vi "Demo_1.vi"() -> ()   [LabVIEW 2014]
uses:
  TypeDefs/Boolean&NumericData.ctl
  <vilib>/Utility/miscctls.llb/LVRowAndColumnTypeDef.ctl
  TypeDefs/LogicParsedExpression.ctl
  TypeDefs/Variable State.ctl
  <vilib>/Utility/file.llb/Read From Spreadsheet File (string).vi
panel:
  in  "Start":bool
  in  "Open Cfg":bool
  in  "Save Cfg":bool
  in  "New Cfg":bool
  in  "Secuencia de Ciclo de Medición":string[][](table)
  in  "Close Seq":bool
  out "Tab Control":enum32{"HOME", "CONFIG.", "CICLO"}(tab)
  out "Editor de Programas Ind":string[][](table)
  in  "Editor de Programas Ctl":string[][](table)
  in  "Diseño":string
  in  "Cód. Prog.":i32
  in  "Autor":string
  in  "Nombre Programa":string
  in  "Descripción":string
  in  "Pieza":i32
  in  "Operación":i32
  in  "Tipo de Programa":enum16{"CAP", "Engranometro"}(ring)
  in  "Secuencia Ciclo":bool
  in  "Secuencia de Ciclo de Medición":string[][](table)
  out "Estado":string
  in  "Angle":sgl(knob) scale=-720.0..720.0
  in  "Cluster":T1
  in  "CICLO":bool
  in  "CONFIG.":bool
  in  "HOME":bool
  in  "Ruta de Sec":path
  in  "Logic Variable Data":T2
  out "error out":errorcluster
  in  "error in (no error)":errorcluster
  # "DEMO Modulo Secuencial"
  # "Programa de Medición"
  # "Instrucciones de Uso"
  # "- Panel Configuración-\n1. Crear Nuevo Configuración o Abrir una ya existente \n\n- Panel Driver -\n1. En la lista desplegable se pueden visualizar y selecciona\n2. Una vez seleccionado un Proceso se puede \n3. Para acceder a su panel de configuración \n\n- CONECTAR -\n1. Una vez definida la configuración de Drivers que uno desea, al presionar \"Conectar >\" se establec\n\n- Panel Dispositivos Conectados -\n1. Una vez conectados los dispositivos se podrá seleccionar cada Dispositivo que esté \n\n- DESCONECTAR -\n1. Una vez que desee terminar con la adquisición, debe presionar \"Desconectar\nsino la aplicación devolverá error."
  # "Editor de Programa de Medición"
  # "Secuencia de Ciclo de Medición"
  # "Entradas Numeradas"
  # "Encoder"
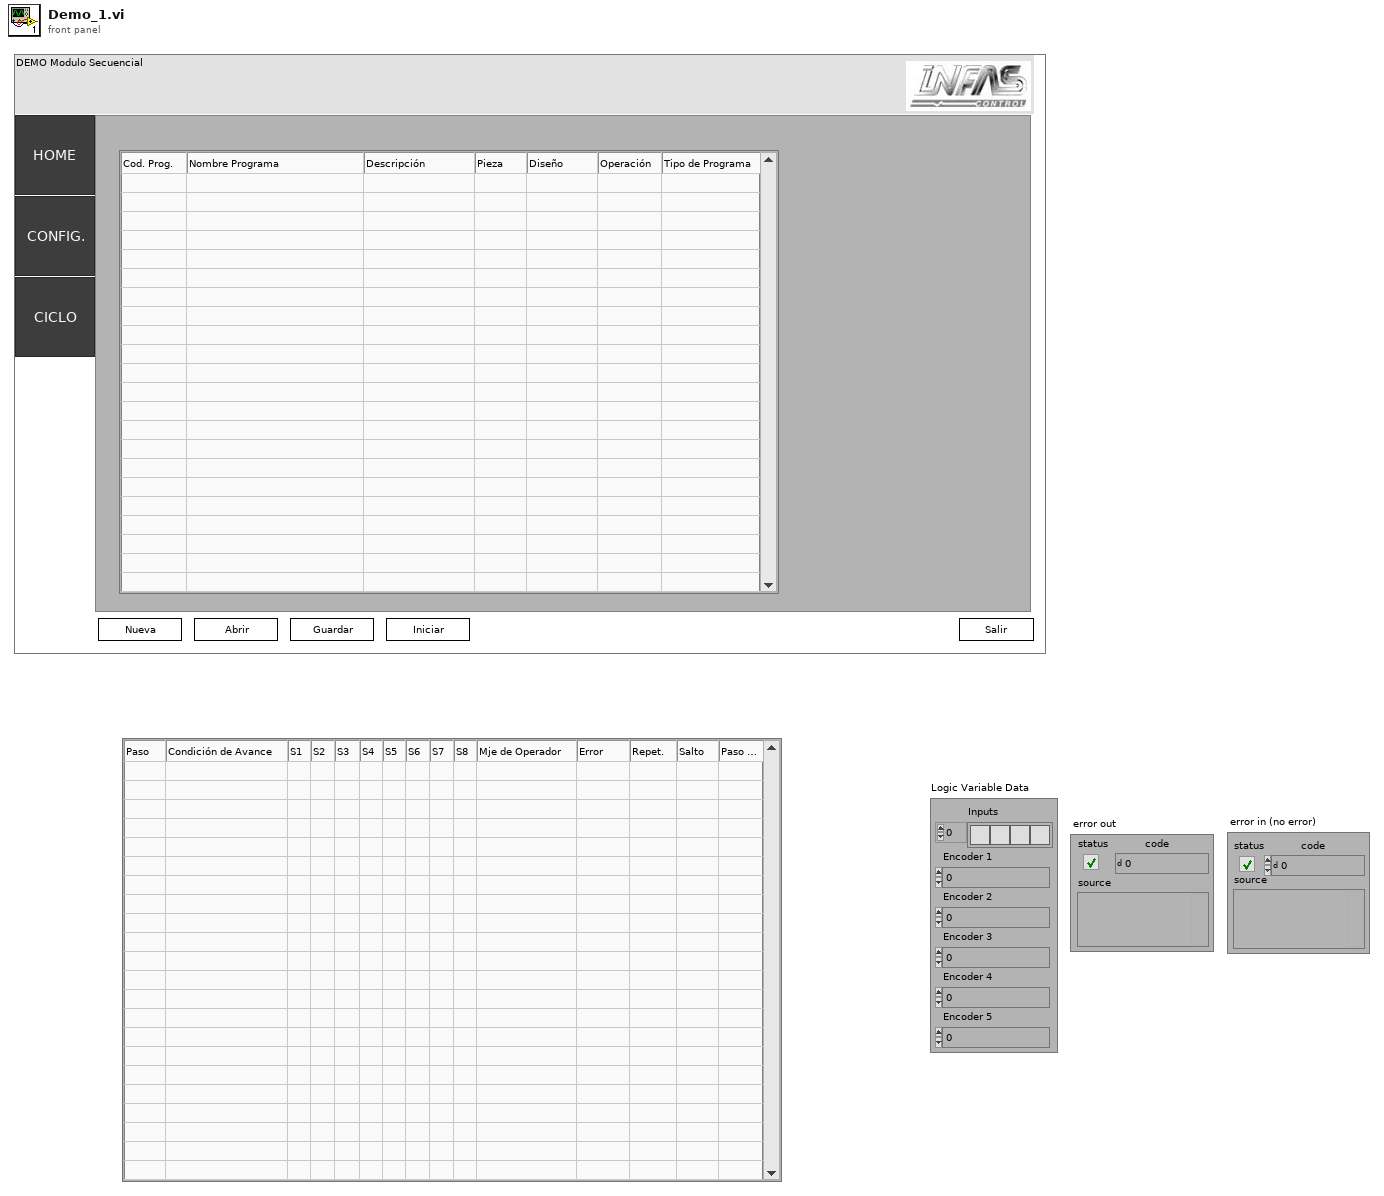
[diagram p1: front panel]
types:
  T1 = cluster{"Boolean 2":bool, "Boolean 1":bool, "Boolean 3":bool, "Boolean 4":bool, "Boolean 5":bool, "Boolean 6":bool, "Boolean 7":bool, "Boolean 8":bool, "Boolean 9":bool, "Boolean 10":bool, "Boolean 11":bool, "Boolean 12":bool}
  T2 = typedef "Boolean&NumericData.ctl" = cluster{"Inputs":bool[], "Encoder 1":sgl, "Encoder 2":sgl, "Encoder 3":sgl, "Encoder 4":sgl, "Encoder 5":sgl}
  T3 = typedef "Variable State.ctl" = cluster{"I":bool[], "P":bool[], "N":bool[], "T":bool[], "X":bool[], "Timer":u32[], "Wait":u32, "Wait?":bool}
  T4 = typedef "LogicParsedExpression.ctl" = cluster{"RPN ":string[], "Variables":string[], "Ctes":string[], "Formula":string, "Message":string}
  T5 = typedef "LVRowAndColumnTypeDef.ctl" = cluster{"Row":i32, "Column":i32}
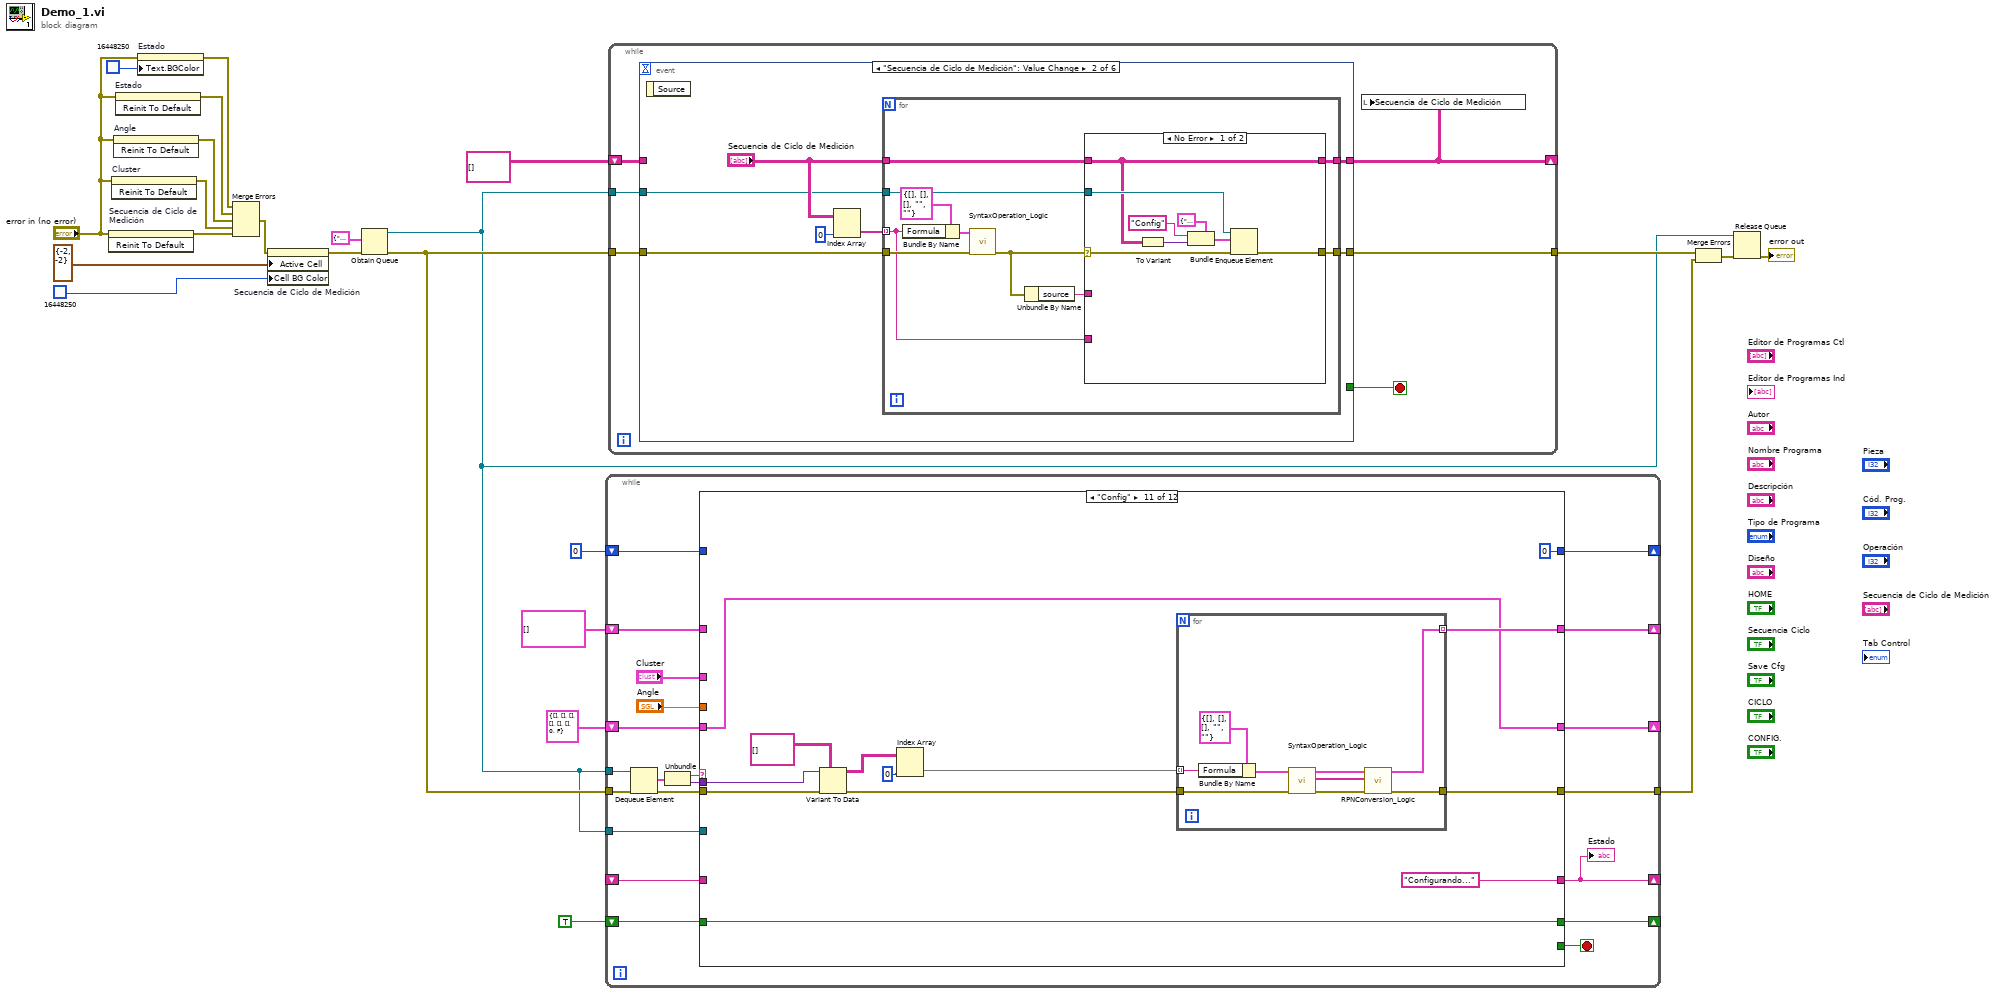
[diagram p0: block diagram]
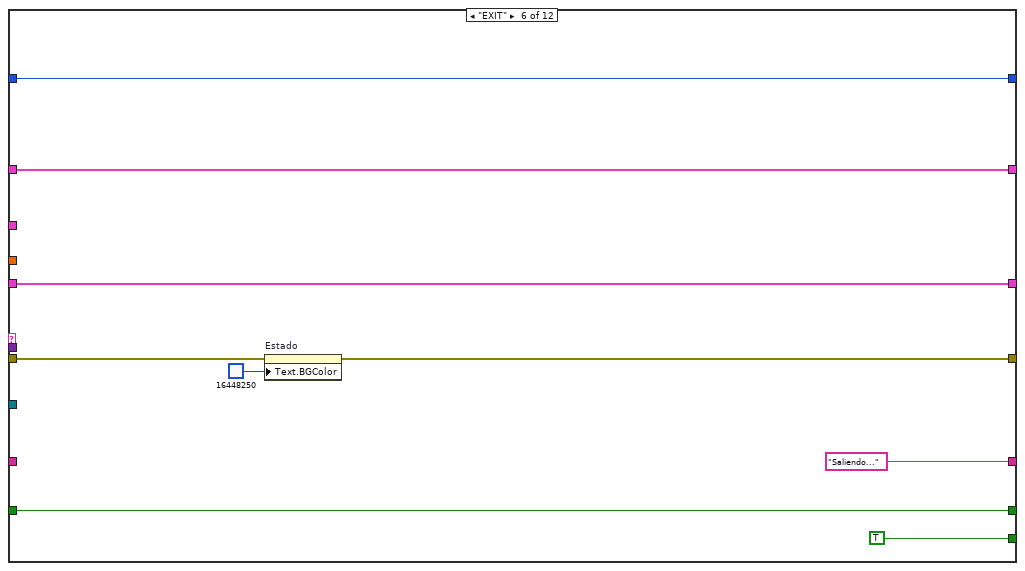
[diagram p7: hidden frame]
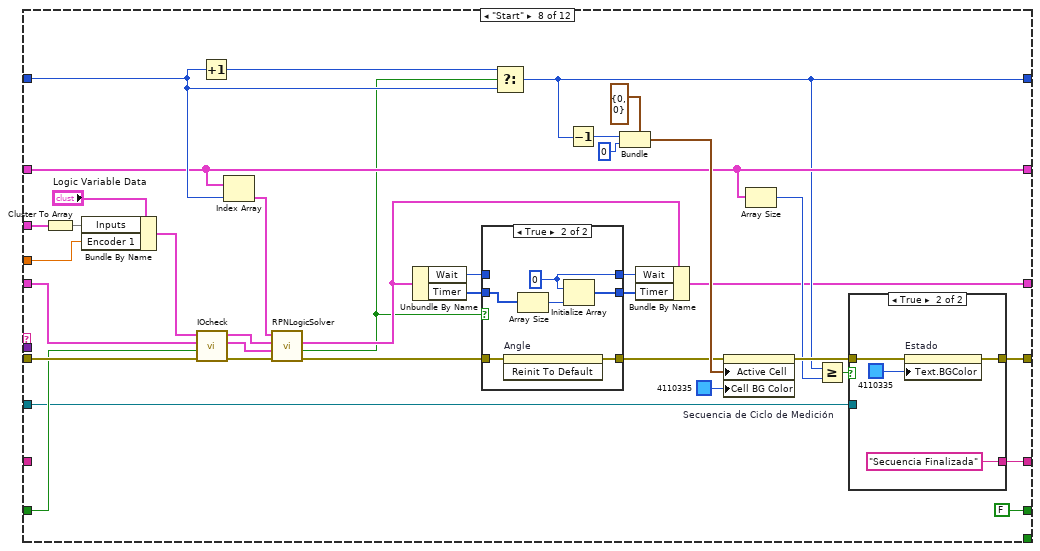
[diagram p9: hidden frame]
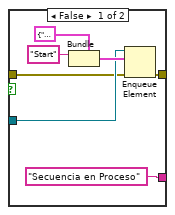
[diagram p11: hidden frame]
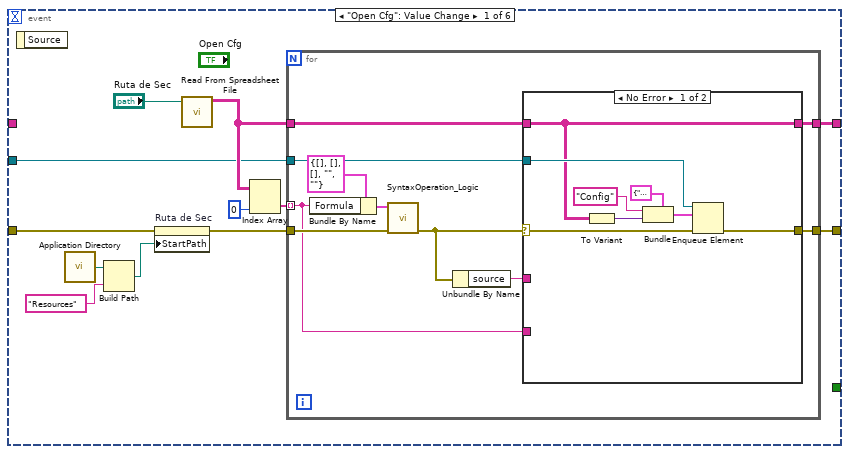
[diagram p15: hidden frame]
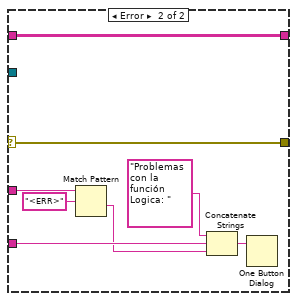
[diagram p16: hidden frame]
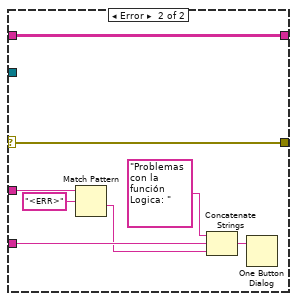
[diagram p17: hidden frame]
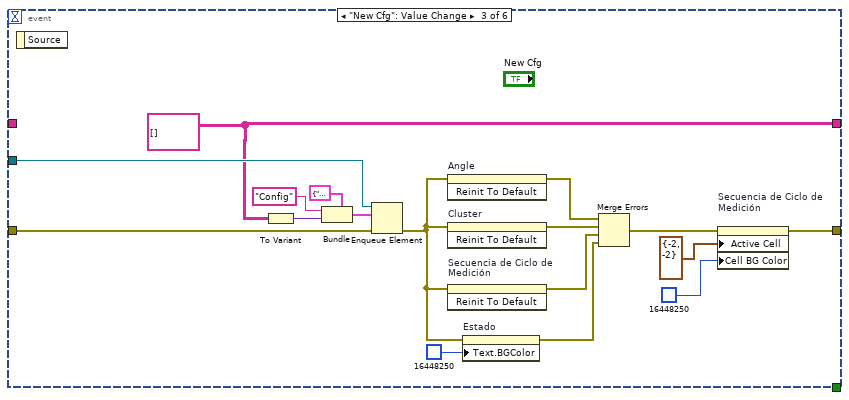
[diagram p18: hidden frame]
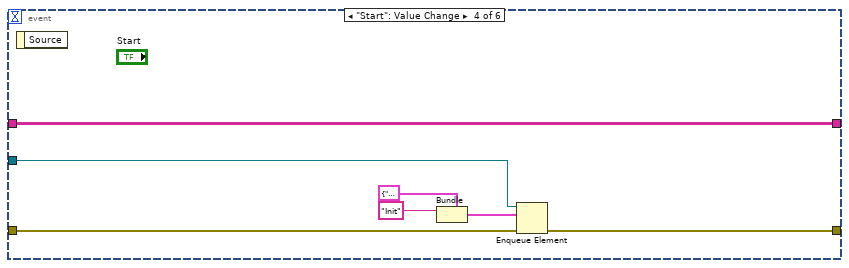
[diagram p19: hidden frame]
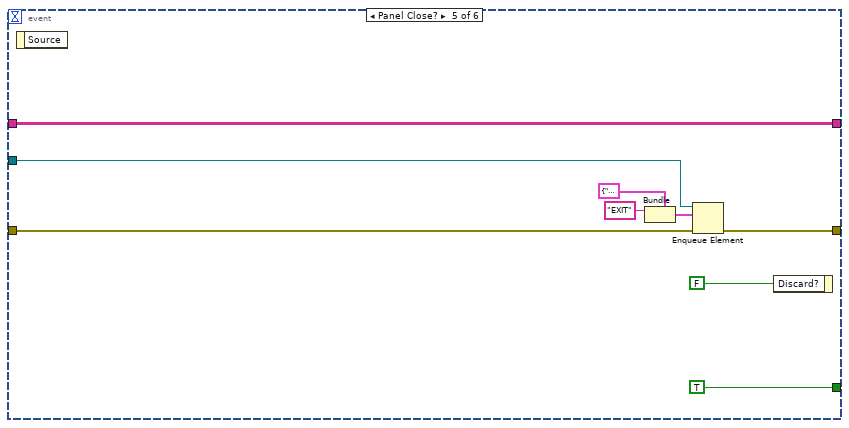
[diagram p20: hidden frame]
diagram:
  n1 = invoke on="Secuencia de Ciclo de Medición" class="Tbl (strict)" method="Reinit To Default"(error in="error in (no error)") -> (error out=w13:errorcluster)  [unwired: 2 in, 2 out]
  n2 = invoke on="Cluster" class="Clust (strict)" method="Reinit To Default"(error in="error in (no error)") -> (error out=w11:errorcluster)  [unwired: 2 in, 2 out]
  n3 = invoke on="Angle" class="Knob (strict)" method="Reinit To Default"(error in="error in (no error)") -> (error out=w5:errorcluster)  [unwired: 2 in, 2 out]
  n4 = invoke on="Estado" class="Str" method="Reinit To Default"(error in="error in (no error)") -> (error out=w4:errorcluster)  [unwired: 2 in, 2 out]
  n5 = property on="Estado" class="Str"(error in="error in (no error)", "Text.BGColor"=u32 16448250) -> (error out=w1:errorcluster)  [unwired: 1 in, 1 out]
  n6 = Merge Errors(w1, w4, w5, w11, w13) -> (w12:errorcluster)
  n7 = property on="Secuencia de Ciclo de Medición" class="Tbl (strict)"(error in=w12, "Active Cell"=T5 {"Row"=-2, "Column"=-2} ("Active Cell:Active Cell"), "Cell BG Color"=u32 16448250) -> (error out=w19:errorcluster)  [unwired: 1 in, 1 out]
  n8 = Obtain Queue(element data type=cluster{string, variant} {"", variant}, error in (no error)=w19) -> (queue out=w6:refnum<queue>, error out=w18:errorcluster)  [unwired: 3 in, 1 out]
  n9 = while {
    tunnel: w18 -> [w43]
    tunnel: [w44] -> w16
    tunnel: w6 -> [w42]
    shift-right: [w35] -> _
    shift-left: T4[] [] -> [w36]
    shift-right: [w33] -> _
    shift-left: T3 {"I"=[], "P"=[], "N"=[], "T"=[], "X"=[], "Timer"=[], "Wait"=0, "Wait?"=FALSE} ("Variable State") -> [w34]
    shift-right: [w31] -> _
    shift-left: TRUE ("First call?") -> [w32]
    shift-right: [w30] -> _
    shift-left: 0 -> [w29]
    tunnel: w6 -> [w28]
    shift-right: [w25] -> _
    shift-left: _ -> [w24]
    stop <- w37 stop-if-true
    n10 = Dequeue Element(queue=w42, error in (no error)=w43) -> (element=w41:cluster{string, variant}, error out=w38:errorcluster)  [unwired: 1 in, 2 out]
    n11 = Unbundle(w41) -> (w40:string, w39:variant)
    n12 = case shown="\"Config\"" w40 {
      tunnel: [w47 w52 w59 w65 w71 w75 w89 w107 w149 w155 w164 w183] -> w44
      tunnel: w38 -> [w47 w52 w59 w65 w71 w76 w89 w126 w149 w155 w171 w183]
      tunnel: w39 -> [_ _ _ _ _ _ _ _ _ _ w170 _]
      tunnel: [_ _ _ _ _ TRUE _ _ _ _ _ _] -> w37
      tunnel: w36 -> [w49 w54 w61 w67 w73 w82 w88 w105 w151 w157 _ w185]
      tunnel: [w49 w54 w61 w67 w73 w82 w88 w105 w151 w157 w163 w185] -> w35
      tunnel: w34 -> [w48 w53 w60 w66 w72 w80 w87 w125 w150 w156 w161 w184]
      tunnel: [w48 w53 w60 w66 w72 w80 w87 w93 w150 w156 w161 w184] -> w33
      tunnel: w32 -> [w45 w56 w57 w63 w69 w81 w86 w124 w147 w153 w162 w181]
      tunnel: [w45 w56 w57 w63 w69 w81 w86 FALSE ("First call?") w147 w153 w162 w181] -> w31
      tunnel: [w50 w55 w62 w68 w74 w79 w85 w103 w152 w158 0 w186] -> w30
      tunnel: w29 -> [w50 w55 w62 w68 w74 w79 w85 w110 w152 w158 _ w186]
      tunnel: w28 -> [_ _ _ _ _ _ _ w109 _ _ _ _]
      tunnel: "Cluster" -> [_ _ _ _ _ _ _ w100 _ _ _ _]
      tunnel: "Angle" -> [_ _ _ _ _ _ _ w99 _ _ _ _]
      tunnel: [w46 w51 w58 w64 w70 "Saliendo..." w84 w94 w148 w154 "Configurando..." w182] -> w25
      tunnel: w24 -> [w46 w51 w58 w64 w70 _ w84 _ w148 w154 _ w182]
      frame "----LOOP----" {
        # "Bloque que adminte futuras configuraciones al inicio."
      }
      frame Default {
      }
      frame "LOAD" {
      }
      frame "INIT" {
      }
      frame "UPLOAD" {
      }
      frame "EXIT" {
        n13 = property on="Estado" class="Str"(error in=w76, "Text.BGColor"=u32 16448250) -> (error out=w75:errorcluster)  [unwired: 1 in, 1 out]
      }
      frame "----ACTION----" {
      }
      frame "Start" {
        n14 = Cluster To Array(cluster=w100) -> (array=w112:bool[])
        n15 = Bundle By Name(cluster="Logic Variable Data", "Inputs"=w112, "Encoder 1"=w99) -> (w113:T2)
        n16 = call "IOcheck.vi"("error in (no error)"=w126, "First call?"=w124, "Variable State"=w125, "Logic Variable Data"=w113) -> ("error out"=w116:errorcluster, "Variable State Out"=w117:T3, "Logic Variable Data Out"=w118:T2)  [unwired: 5 in]
        n17 = Increment(x=w110) -> (x+1=w115:i32)
        n18 = Index Array(array=w105, index=w110) -> (element=w111:T4)
        n19 = call "RPNLogicSolver.vi"("error in"=w116, "Variable State"=w117, "Logic Variable Data Out"=w118, "Logic Parsed Expression"=w111) -> ("error out"=w96:errorcluster, "Logical Operation Out"=w92:bool, "Variable State Out"=w101:T3)  [unwired: 4 in, 1 out]
        n20 = Unbundle By Name(w101) -> ("Wait"=w90:u32, "Timer"=w97:u32[])
        n21 = case shown="True" w92 {
          tunnel: [w129 w134] -> w98
          tunnel: w97 -> [w129 w133]
          tunnel: w96 -> [w128 w132]
          tunnel: [w128 w131] -> w95
          tunnel: [w127 w130] -> w91
          tunnel: w90 -> [w127 _]
          frame False {
          }
          frame True {
            w130 = u32 0 ("element")
            n22 = invoke on="Angle" class="Knob (strict)" method="Reinit To Default"(error in=w132) -> (error out=w131:errorcluster)  [unwired: 2 in, 2 out]
            n23 = Array Size(array=w133) -> (size(s)=w135:i32)
            n24 = Initialize Array(w130, w135) -> (w134:u32[])
          }
        }
        n25 = Select(t=w115, s=w92, f=w110) -> (s? t:f=w103:i32)
        n26 = Decrement(x=w103) -> (x-1=w102:i32)
        n27 = Bundle(cluster=T5 {"Row"=0, "Column"=0} ("Active Cell:Active Cell"), "Row"=w102, "Column"=0 ("Row")) -> (w119:T5)
        n28 = Bundle By Name(cluster=w101, "Wait"=w91, "Timer"=w98) -> (w93:T3)
        n29 = property on="Secuencia de Ciclo de Medición" class="Tbl (strict)"(error in=w95, "Active Cell"=w119, "Cell BG Color"=u32 4110335) -> (error out=w108:errorcluster)  [unwired: 1 in, 1 out]
        n30 = Array Size(array=w105) -> (size(s)=w104:i32)
        n31 = Greater Or Equal?(x=w103, y=w104) -> (x >= y?=w106:bool)
        n32 = case shown="True" w106 {
          tunnel: w109 -> [w139 _]
          tunnel: w108 -> [w138 w145]
          tunnel: [w137 w143] -> w107
          tunnel: ["Secuencia en Proceso" "Secuencia Finalizada"] -> w94
          frame False {
            n33 = Bundle(cluster=cluster{string, variant} {"", variant}, "Start") -> (w142:cluster{string, variant})  [unwired: 1 in]
            n34 = Enqueue Element(queue=w139, element=w142, error in (no error)=w138) -> (error out=w137:errorcluster)  [unwired: 1 in, 2 out]
          }
          frame True {
            n35 = property on="Estado" class="Str"(error in=w145, "Text.BGColor"=u32 4110335) -> (error out=w143:errorcluster)  [unwired: 1 in, 1 out]
          }
        }
      }
      frame "----UTILITY----" {
      }
      frame "Config:Set" {
      }
      frame "Config" {
        n36 = Variant To Data(error in=w171, type=string[][] [] ("Secuencia de Ciclo de Medición"), Variant=w170) -> (data=w167:string[][], error out=w165:errorcluster)
        n37 = Index Array(array=w167, index (col)=0 ("index (row)")) -> (element=w166:string[])  [unwired: 1 in]
        n38 = for {
          tunnel: w166 -> [w176] mode=indexing
          tunnel: w165 -> [w175]
          tunnel: [w174] -> w164
          tunnel: [w173] -> w163 mode=indexing
          n39 = Bundle By Name(cluster=T4 {"RPN "=[], "Variables"=[], "Ctes"=[], "Formula"="", "Message"=""} ("Logical Parsed Expression Out"), "Formula"=w176) -> (w177:T4)
          n40 = call "SyntaxOperation_Logic.vi"("error in (no error)"=w175, "Logical Parsed Expression"=w177) -> ("error out"=w178:errorcluster, "Token"=w180:string[], "Logical Parsed Expression Out"=w179:T4)  [unwired: 6 in, 1 out]
          n41 = call "RPNConversion_Logic.vi"("error in"=w178, "Token"=w180, "Logical Parsed Expression"=w179) -> ("error out"=w174:errorcluster, "Logical Parsed Expression Out"=w173:T4)  [unwired: 7 in]
        }
      }
      frame "Config:Get" {
      }
    }
    "Estado" <- w25
  }
  n42 = while {
    tunnel: w18 -> [w191]
    tunnel: [w190] -> w15
    shift-right: [w187] -> _
    shift-left: string[][] [] ("Secuencia de Ciclo de Medición") -> [w192]
    tunnel: w6 -> [w188]
    stop <- w189 stop-if-true
    n43 = event shown="[1] \"Secuencia de Ciclo de Medición\": Value Change" {
      selector: _ -> [_ _ _ _ _ _]
      dyn-events: _ -> [_ _ _ _ _ _]
      timeout: _ -> [_ _ _ _ _ _]
      tunnel: w192 -> [_ _ _ w287 w296 w303]
      tunnel: w191 -> [w194 w233 w275 w284 w292 w299]
      tunnel: [w201 w234 w267 w283 w291 w298] -> w190
      tunnel: [w202 w231 w274 w287 w296 w303] -> w187
      tunnel: [_ _ _ _ TRUE ("Discard?") TRUE ("Discard?")] -> w189
      tunnel: w188 -> [w199 w232 w276 w282 w288 w297]
      event "Open Cfg": Value Change {
        n44 = event-data() -> ()  [unwired: 1 in, 1 out]
        n45 = call <vilib>:"Application Directory.vi"() -> ("Application Directory"=w197:path)
        n46 = Build Path(base path=w197, name or relative path="Resources") -> (appended path=w195:path)
        n47 = property on="Ruta de Sec" class="Path"(error in=w194, "StartPath"=w195) -> (error out=w193:errorcluster)  [unwired: 1 in, 1 out]
        n48 = call-poly <vilib>:"Read From Spreadsheet File.vi"("file path (dialog if empty)"="Ruta de Sec") -> ("all rows"=w200:string[][])  [unwired: 6 in, 4 out]
        n49 = Index Array(array=w200, index (col)=0 ("disabled index (col)")) -> (element=w203:string[])  [unwired: 1 in]
        n50 = for {
          tunnel: w203 -> [w205] mode=indexing
          tunnel: w200 -> [w213]
          tunnel: [w212] -> w201
          tunnel: w193 -> [w211]
          tunnel: w199 -> [w210]
          tunnel: [w209] -> w202
          n51 = Bundle By Name(cluster=T4 {"RPN "=[], "Variables"=[], "Ctes"=[], "Formula"="", "Message"=""} ("Logical Parsed Expression"), "Formula"=w205) -> (w206:T4)
          n52 = call "SyntaxOperation_Logic.vi"("error in (no error)"=w211, "Logical Parsed Expression"=w206) -> ("error out"=w208:errorcluster)  [unwired: 6 in, 3 out]
          n53 = Unbundle By Name(w208) -> ("source"=w207:string)
          n54 = case shown="No Error" w208 {
            selector: w208 -> [w215 w230]
            tunnel: w213 -> [w216 w229]
            tunnel: [w218 w230] -> w212
            tunnel: w210 -> [w217 _]
            tunnel: [w216 w229] -> w209
            tunnel: w207 -> [_ w228]
            tunnel: w205 -> [_ w224]
            frame No Error {
              n55 = To Variant(anything=w216) -> (Variant=w221:variant)
              n56 = Bundle(cluster=cluster{string, variant} {"", variant}, "Config", w221) -> (w219:cluster{string, variant})
              n57 = Enqueue Element(queue=w217, element=w219, error in (no error)=w215) -> (error out=w218:errorcluster)  [unwired: 1 in, 2 out]
            }
            frame Error {
              n58 = Match Pattern(string=w228, regular expression="<ERR>") -> (after substring=w223:string)  [unwired: 1 in, 3 out]
              n59 = Concatenate Strings("Problemas con la función Logica: " ("string"), w224, w223) -> (w226:string)
              n60 = One Button Dialog(message=w226) -> ()  [unwired: 1 in, 1 out]
            }
          }
        }
      }
      event "Secuencia de Ciclo de Medición": Value Change {
        n61 = event-data() -> ()  [unwired: 1 in, 1 out]
        n62 = Index Array(array="Secuencia de Ciclo de Medición", index (col)=0 ("disabled index (col)")) -> (element=w236:string[])  [unwired: 1 in]
        n63 = for {
          tunnel: w236 -> [w238] mode=indexing
          tunnel: "Secuencia de Ciclo de Medición" -> [w246]
          tunnel: [w245] -> w234
          tunnel: w233 -> [w244]
          tunnel: w232 -> [w243]
          tunnel: [w242] -> w231
          n64 = Bundle By Name(cluster=T4 {"RPN "=[], "Variables"=[], "Ctes"=[], "Formula"="", "Message"=""} ("Logical Parsed Expression"), "Formula"=w238) -> (w239:T4)
          n65 = call "SyntaxOperation_Logic.vi"("error in (no error)"=w244, "Logical Parsed Expression"=w239) -> ("error out"=w241:errorcluster)  [unwired: 6 in, 3 out]
          n66 = Unbundle By Name(w241) -> ("source"=w240:string)
          n67 = case shown="No Error" w241 {
            selector: w241 -> [w248 w263]
            tunnel: w246 -> [w249 w262]
            tunnel: [w251 w263] -> w245
            tunnel: w243 -> [w250 _]
            tunnel: [w249 w262] -> w242
            tunnel: w240 -> [_ w261]
            tunnel: w238 -> [_ w257]
            frame No Error {
              n68 = To Variant(anything=w249) -> (Variant=w254:variant)
              n69 = Bundle(cluster=cluster{string, variant} {"", variant}, "Config", w254) -> (w252:cluster{string, variant})
              n70 = Enqueue Element(queue=w250, element=w252, error in (no error)=w248) -> (error out=w251:errorcluster)  [unwired: 1 in, 2 out]
            }
            frame Error {
              n71 = Match Pattern(string=w261, regular expression="<ERR>") -> (after substring=w256:string)  [unwired: 1 in, 3 out]
              n72 = Concatenate Strings("Problemas con la función Logica: " ("string"), w257, w256) -> (w259:string)
              n73 = One Button Dialog(message=w259) -> ()  [unwired: 1 in, 1 out]
            }
          }
        }
      }
      event "New Cfg": Value Change {
        w274 = string[][] [] ("Secuencia de Ciclo de Medición")
        n74 = event-data() -> ()  [unwired: 1 in, 1 out]
        n75 = To Variant(anything=w274) -> (Variant=w279:variant)
        n76 = Bundle(cluster=cluster{string, variant} {"", variant}, "Config", w279) -> (w277:cluster{string, variant})
        n77 = Enqueue Element(queue=w276, element=w277, error in (no error)=w275) -> (error out=w264:errorcluster)  [unwired: 1 in, 2 out]
        n78 = invoke on="Angle" class="Knob (strict)" method="Reinit To Default"(error in=w264) -> (error out=w268:errorcluster)  [unwired: 2 in, 2 out]
        n79 = invoke on="Cluster" class="Clust (strict)" method="Reinit To Default"(error in=w264) -> (error out=w269:errorcluster)  [unwired: 2 in, 2 out]
        n80 = invoke on="Secuencia de Ciclo de Medición" class="Tbl (strict)" method="Reinit To Default"(error in=w264) -> (error out=w271:errorcluster)  [unwired: 2 in, 2 out]
        n81 = property on="Estado" class="Str"(error in=w264, "Text.BGColor"=u32 16448250) -> (error out=w265:errorcluster)  [unwired: 1 in, 1 out]
        n82 = Merge Errors(w268, w269, w271, w265) -> (w270:errorcluster)
        n83 = property on="Secuencia de Ciclo de Medición" class="Tbl (strict)"(error in=w270, "Active Cell"=T5 {"Row"=-2, "Column"=-2} ("Active Cell:Active Cell"), "Cell BG Color"=u32 16448250) -> (error out=w267:errorcluster)  [unwired: 1 in, 1 out]
      }
      event "Start": Value Change {
        n84 = event-data() -> ()  [unwired: 1 in, 1 out]
        n85 = Bundle(cluster=cluster{string, variant} {"", variant}, "Init") -> (w286:cluster{string, variant})  [unwired: 1 in]
        n86 = Enqueue Element(queue=w282, element=w286, error in (no error)=w284) -> (error out=w283:errorcluster)  [unwired: 1 in, 2 out]
      }
      event Panel Close? {
        n87 = event-data() -> ()  [unwired: 1 in, 1 out]
        n88 = Bundle(cluster=cluster{string, variant} {"", variant}, "EXIT") -> (w290:cluster{string, variant})  [unwired: 1 in]
        n89 = Enqueue Element(queue=w288, element=w290, error in (no error)=w292) -> (error out=w291:errorcluster)  [unwired: 1 in, 2 out]
        n90 = event-data("Discard?"=FALSE) -> ()  [unwired: 1 in, 1 out]
      }
      event "Close Seq": Value Change {
        n91 = event-data() -> ()  [unwired: 1 in, 1 out]
        n92 = Bundle(cluster=cluster{string, variant} {"", variant}, "EXIT") -> (w302:cluster{string, variant})  [unwired: 1 in]
        n93 = Enqueue Element(queue=w297, element=w302, error in (no error)=w299) -> (error out=w298:errorcluster)  [unwired: 1 in, 2 out]
      }
    }
    n94 = local write "Secuencia de Ciclo de Medición"(w187) -> ()
  }
  n95 = Merge Errors(w15, w16) -> (w14:errorcluster)
  n96 = Release Queue(queue=w6, error in (no error)=w14) -> (error out=→"error out":errorcluster)  [unwired: 1 in, 2 out]
